vi "Get Table Position.vi"(8 "error in (no error)":errorcluster, 11 "XRay Table in":refnum<class "XRay Table.lvclass">) -> (0 "error out":errorcluster, 1 "Y Position":dbl, 2 "X Position":dbl, 3 "XRay Table out":refnum<class "XRay Table.lvclass">, 4 "Pos Changed":bool, 5 "Table Rotation":dbl)   [LabVIEW 2026, in "XRay Table.lvclass"]
uses:
  XRay Table.lvclass
  XRay Table.lvclass/XRay Table.ctl
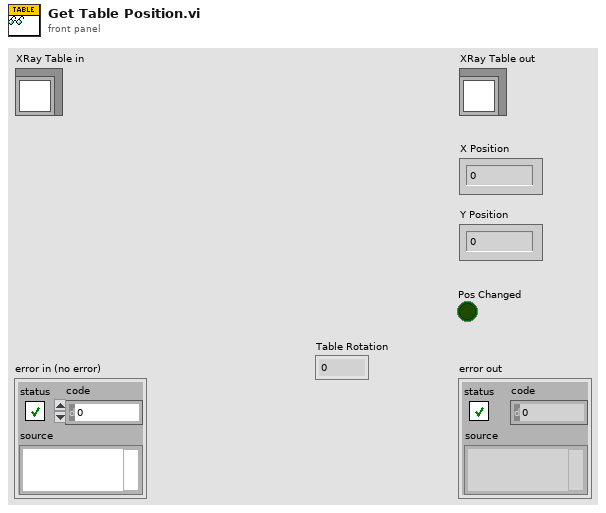
[diagram p1: front panel]
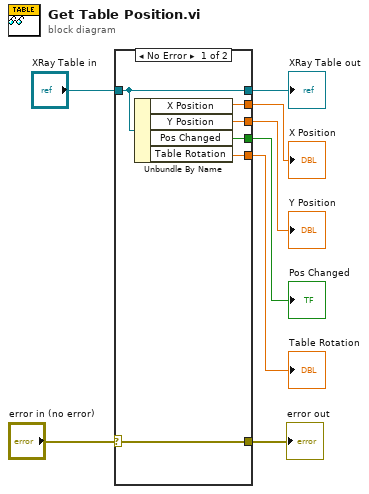
[diagram p0: block diagram]
diagram:
  n1 = case shown="No Error" "error in (no error)" {
    selector: "error in (no error)" -> [w14 w15]
    tunnel: [w14 w15] -> w7
    tunnel: [w13 w16] -> w5
    tunnel: "XRay Table in" -> [w13 w16]
    tunnel: [w12 _] -> w4
    tunnel: [w11 _] -> w3
    tunnel: [w10 _] -> w2
    tunnel: [w9 _] -> w1
    frame No Error {
      n2 = Unbundle By Name(w13) -> ("X Position"=w12:dbl, "Y Position"=w11:dbl, "Pos Changed"=w10:bool, "Table Rotation"=w9:dbl)
    }
    frame Error {
    }
  }
  "error out" <- w7
  "XRay Table out" <- w5
  "X Position" <- w4
  "Y Position" <- w3
  "Pos Changed" <- w2
  "Table Rotation" <- w1
